vi "NI 9260 Synchronization 9230 (Host).vi"() -> ()   [LabVIEW 2021]
uses:
  <vilib>/LabVIEW Targets/FPGA/cRIO/shared/nicrio_ModuleControls/nicrio_cRIO-9260_DataRatesRing2.ctl
  <vilib>/LabVIEW Targets/FPGA/cRIO/shared/nicrio_ModuleControls/nicrio_cRIO-9230_DataRatesRing2.ctl
  <vilib>/FPGAPlugInAG/cRIO-9053/niLvFpga_Open_cRIO-9053.vi
  <vilib>/rvi/interface/common/dynamic/niFpgaDynamicAddResources.vi
  <vilib>/Utility/error.llb/Error Cluster From Error Code.vi
  <vilib>/rvi/errors/niLvFpgaAdjustHostInterfaceError.vi
  <vilib>/rvi/interface/common/niFpgaWaitOnOcc.vi
  <vilib>/FPGAPlugInAG/Dynamic/niLvFpga_Run_Dynamic.vi
  <vilib>/FPGAPlugInAG/Dynamic/niLvFpga_Close_Dynamic.vi
  <vilib>/rvi/interface/nirviOpenFPGA/nirviOpenFPGA.xnode
  FPGA Bitfiles/crio-ni9260_FPGATarget_NI9260Synchroniz_8mHRFd2dl5A.lvbitx
  <vilib>/rvi/interface/nirviReadWriteControl/nirviReadWriteControl.xnode
  <vilib>/rvi/interface/nirviMethod/nirviMethod.xnode
  <vilib>/rvi/interface/nirviCloseFPGA/nirviCloseFPGA.xnode
  <vilib>/rvi/interface/Simulation/niFpgaSimulationCallBeginRW.vi
  <vilib>/FPGAPlugInAG/Dynamic/niLvFpga_WriteFifo_Dynamic.vi
  <vilib>/rvi/errors/niLvFpgaMergeErrorWithErrorCode.vi
  <vilib>/FPGAPlugInAG/Dynamic/niLvFpga_ConfigureFifo_Dynamic.vi
  NiFpgaLv.dll
  <vilib>/FPGAPlugInAG/Dynamic/niLvFpga_ReadFifo_Dynamic.vi
panel:
  out "host rate (ms)":u32=80
  in  "Waveform":T1(ring)=enum."Square Wave"
  in  "NI 9230 Data Rate":T2=10 items=["12.800 kS/s (NI 9230)"=10, "11.378 kS/s (NI 9230)"=36, "10.240 kS/s (NI 9230)"=21, "9.309 kS/s (NI 9230)"=44, "8.533 kS/s (NI 9230)"=14, "7.877 kS/s (NI 9230)"=52, "7.314 kS/s (NI 9230)"=29, "6.827 kS/s (NI 9230)"=60, "6.400 kS/s (NI 9230)"=18, "6.024 kS/s (NI 9230)"=68, "5.689 kS/s (NI 9230)"=37, "5.389 kS/s (NI 9230)"=76, "5.120 kS/s (NI 9230)"=22, "4.876 kS/s (NI 9230)"=84, "4.655 kS/s (NI 9230)"=45, "4.452 kS/s (NI 9230)"=92, "4.267 kS/s (NI 9230)"=26, "4.096 kS/s (NI 9230)"=100, "3.938 kS/s (NI 9230)"=53, "3.657 kS/s (NI 9230)"=30, "3.413 kS/s (NI 9230)"=61, "3.200 kS/s (NI 9230)"=34, "3.012 kS/s (NI 9230)"=69, "2.844 kS/s (NI 9230)"=38, "2.695 kS/s (NI 9230)"=77, "2.560 kS/s (NI 9230)"=42, "2.438 kS/s (NI 9230)"=85, "2.327 kS/s (NI 9230)"=46, "2.226 kS/s (NI 9230)"=93, "2.133 kS/s (NI 9230)"=50, "2.048 kS/s (NI 9230)"=101, "1.969 kS/s (NI 9230)"=54, "1.829 kS/s (NI 9230)"=58, "1.707 kS/s (NI 9230)"=62, "1.600 kS/s (NI 9230)"=66, "1.506 kS/s (NI 9230)"=70, "1.422 kS/s (NI 9230)"=74, "1.347 kS/s (NI 9230)"=78, "1.280 kS/s (NI 9230)"=82, "1.219 kS/s (NI 9230)"=86, "1.164 kS/s (NI 9230)"=90, "1.113 kS/s (NI 9230)"=94, "1.067 kS/s (NI 9230)"=98, "1.024 kS/s (NI 9230)"=102, "0.985 kS/s (NI 9230)"=106]
  in  "NI 9260 Data Rate":T3=4 items=["51.200 kS/s (NI 9260)"=1, "25.600 kS/s (NI 9260)"=2, "17.067 kS/s (NI 9260)"=3, "12.800 kS/s (NI 9260)"=4, "10.240 kS/s (NI 9260)"=5, "8.533 kS/s (NI 9260)"=6, "7.314 kS/s (NI 9260)"=7, "6.400 kS/s (NI 9260)"=8, "5.689 kS/s (NI 9260)"=9, "5.120 kS/s (NI 9260)"=10, "4.654 kS/s (NI 9260)"=11, "4.267 kS/s (NI 9260)"=12, "3.938 kS/s (NI 9260)"=13, "3.657 kS/s (NI 9260)"=14, "3.413 kS/s (NI 9260)"=15, "3.200 kS/s (NI 9260)"=16, "3.012 kS/s (NI 9260)"=17, "2.845 kS/s (NI 9260)"=18, "2.695 kS/s (NI 9260)"=19, "2.560 kS/s (NI 9260)"=20, "2.438 kS/s (NI 9260)"=21, "2.328 kS/s (NI 9260)"=22, "2.226 kS/s (NI 9260)"=23, "2.133 kS/s (NI 9260)"=24, "2.048 kS/s (NI 9260)"=25, "1.969 kS/s (NI 9260)"=26, "1.896 kS/s (NI 9260)"=27, "1.829 kS/s (NI 9260)"=28, "1.765 kS/s (NI 9260)"=29, "1.707 kS/s (NI 9260)"=30, "1.652 kS/s (NI 9260)"=31]
  out "Analog Input":waveform(dbl)[](graph)=[{"t0"=timestamp(0 s since 1904-01-01), "dt"=7.8125e-05, "Y"=array[1024 elements]}, {"t0"=timestamp(0 s since 1904-01-01), "dt"=7.8125e-05, "Y"=array[1024 elements]}]
  out "NI 9230 FIFO Time Out":bool
  in  "Host Loop Rate (ms)":u32=1
  out "NI 9260 FIFO Time Out":bool
  in  "Waveform Settings":T4(array[cluster])=[{"Frequency (Hz)"=800.0, "Amplitude (V)"=2.5, "Offset (V)"=0.0, "Phase (deg)"=0.0}, {"Frequency (Hz)"=800.0, "Amplitude (V)"=2.5, "Offset (V)"=0.0, "Phase (deg)"=0.0}]
  in  "stop":bool
  out "FPGA Error out":errorcluster
  in  "Number of Samples per channel":dbl=1024.0 format="%.4p"
  out "Analog Output":waveform(dbl)[](graph)=[{"t0"=timestamp(0 s since 1904-01-01), "dt"=7.8125e-05, "Y"=array[1024 elements]}, {"t0"=timestamp(0.08 s since 1904-01-01), "dt"=7.8125e-05, "Y"=array[1024 elements]}]
  out "Host Error out":errorcluster
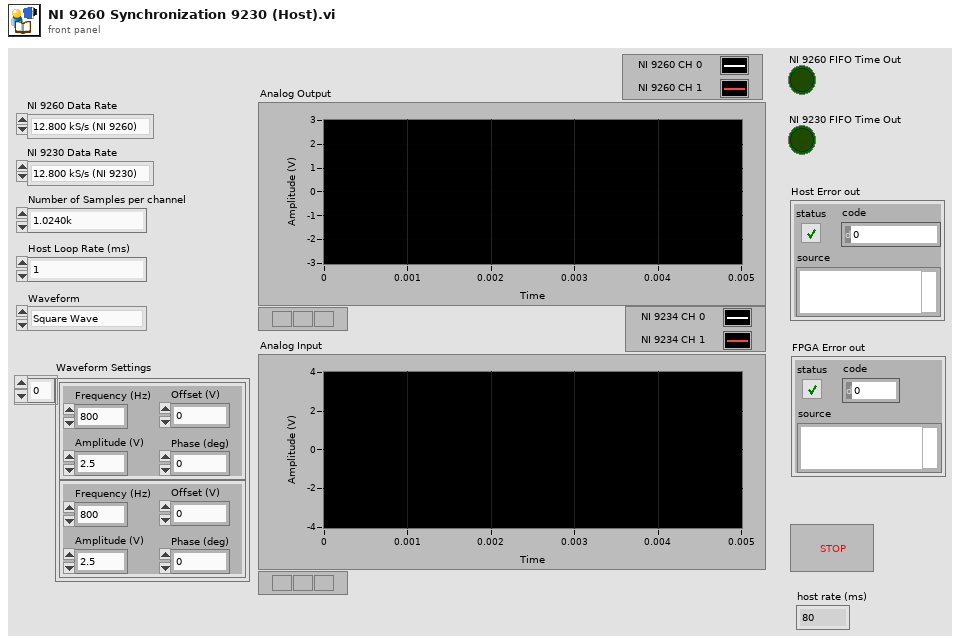
[diagram p1: front panel]
types:
  T1 = enum16{"Sawtooth Wave", "Square Wave", "Sine Wave"}
  T2 = typedef "nicrio_cRIO-9230_DataRatesRing2.ctl" = u8
  T3 = typedef "nicrio_cRIO-9260_DataRatesRing2.ctl" = u8
  T4 = cluster{"Frequency (Hz)":dbl, "Amplitude (V)":dbl, "Offset (V)":dbl, "Phase (deg)":dbl}[]
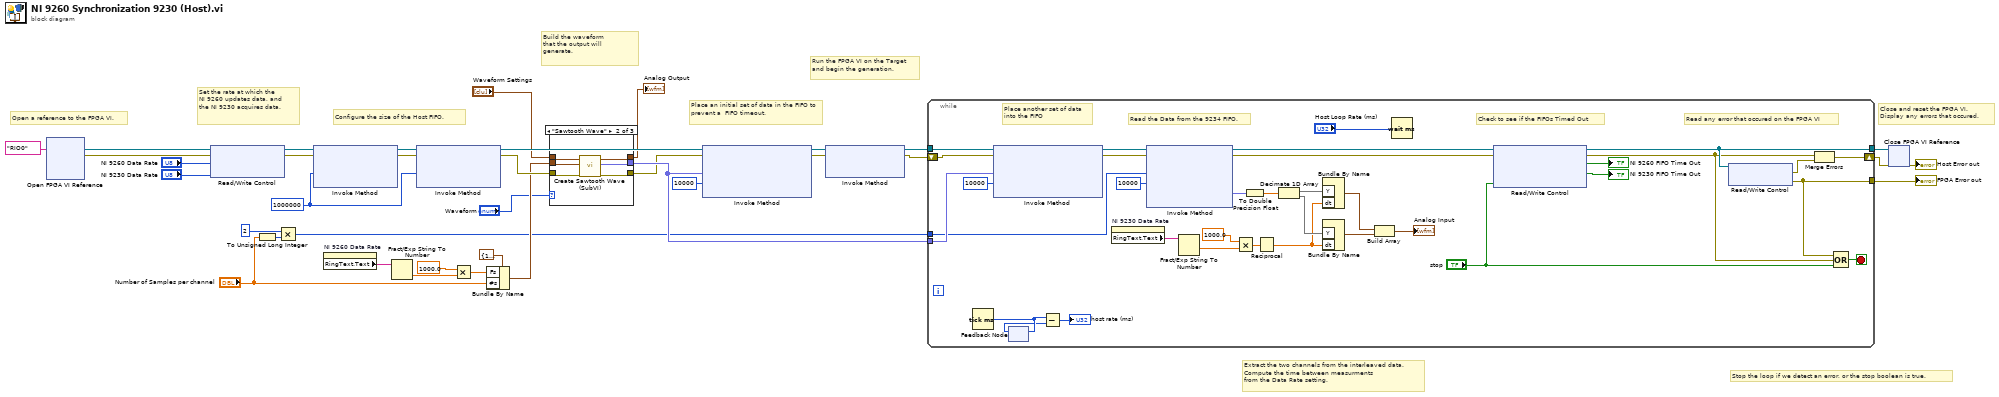
[diagram p0: block diagram]
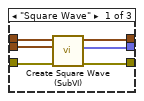
[diagram p2: hidden frame]
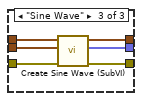
[diagram p3: hidden frame]
diagram:
  w2 = u32 1000000 ("Requested Depth")
  # "Build the waveform \nthat the output will generate."
  # "Extract the two channels from the interleaved data.\nCompute the time between measurments \nfrom the Data Rate setting."
  # "Place an initial set of data in the FIFO to prevent a  FIFO timeout."
  # "Stop the loop if we detect an error, or the stop boolean is true."
  # "Configure the size of the Host FIFO."
  # "Set the rate at which the \nNI 9260 updates data, and\nthe NI 9230 acquires data."
  # "Close and reset the FPGA VI. \nDisplay any errors that occured."
  # "Run the FPGA VI on the Target and begin the generation."
  # "Open a reference to the FPGA VI."
  n1 = xnode "Open FPGA VI Reference"("resource name"=tag "RIO0") -> ("FPGA VI Reference Out"=w34:refnum<k20>, "error out"=w36:errorcluster)  [unwired: 1 in]
  n2 = xnode "Read/Write Control"("FPGA VI Reference In"=w34, "error in"=w36, "NI 9260 Data Rate"="NI 9260 Data Rate", "NI 9230 Data Rate"="NI 9230 Data Rate") -> ("FPGA VI Reference Out"=w16:refnum<k20>, "error out"=w24:errorcluster)
  n3 = To Unsigned Long Integer(number="Number of Samples per channel") -> (unsigned 32bit integer=w29:u32)
  n4 = Multiply(x=u32 2, y=w29) -> (x*y=w3:u32)
  n5 = xnode "Invoke Method"("FPGA VI Reference In"=w16, "error in"=w24, "Requested Depth"=w2) -> ("FPGA VI Reference Out"=w15:refnum<k20>, "error out"=w17:errorcluster)  [unwired: 1 out]
  n6 = property on="NI 9260 Data Rate" class="Ring (strict)"() -> ("RingText.Text"=w5:string)  [unwired: 2 in, 2 out]
  n7 = Fract/Exp String To Number(string=w5) -> (number=w32:dbl)  [unwired: 3 in, 1 out]
  n8 = xnode "Invoke Method"("FPGA VI Reference In"=w15, "error in"=w17, "Requested Depth"=w2) -> ("FPGA VI Reference Out"=w26:refnum<k20>, "error out"=w14:errorcluster)  [unwired: 1 out]
  n9 = Multiply(x=1000.0, y=w32) -> (x*y=w21:dbl)
  n10 = Bundle By Name(cluster=cluster{"Fs":dbl, "#s":dbl} {"Fs"=1000.0, "#s"=1000.0} ("sampling info"), "Fs"=w21, "#s"="Number of Samples per channel") -> (w12:cluster{"Fs":dbl, "#s":dbl})
  n11 = case shown="\"Sawtooth Wave\"" "Waveform" {
    tunnel: w14 -> [w40 w46 w54]
    tunnel: "Waveform Settings" -> [w42 w48 w53]
    tunnel: w12 -> [w41 w47 w52]
    tunnel: [w37 w43 w51] -> w11
    tunnel: [w39 w44 w50] -> w10
    tunnel: [w38 w45 w49] -> w8
    frame "Square Wave" {
      n12 = call "Create Square Wave (SubVI).vi"("error in (no error)"=w40, "sampling info"=w41, "Sine Waveform Settings"=w42) -> ("error out"=w39:errorcluster, "FXP Sinewave"=w37:fxp<+/-,24,4>[], "Voltage Output Waveform"=w38:waveform(dbl)[])  [unwired: 6 in]
    }
    frame "Sawtooth Wave" {
      n13 = call "Create Sawtooth Wave (SubVI).vi"("error in (no error)"=w46, "sampling info"=w47, "Sine Waveform Settings"=w48) -> ("error out"=w44:errorcluster, "FXP Sinewave"=w43:fxp<+/-,24,4>[], "Voltage Output Waveform"=w45:waveform(dbl)[])  [unwired: 6 in]
    }
    frame "Sine Wave" {
      n14 = call "Create Sine Wave (SubVI).vi"("error in (no error)"=w54, "sampling info"=w52, "Sine Waveform Settings"=w53) -> ("error out"=w50:errorcluster, "FXP Sinewave"=w51:fxp<+/-,24,4>[], "Voltage Output Waveform"=w49:waveform(dbl)[])  [unwired: 6 in]
    }
  }
  "Analog Output" <- w8
  n15 = xnode "Invoke Method"("FPGA VI Reference In"=w26, "error in"=w10, "Data"=w11, "Timeout (ms)"=10000) -> ("FPGA VI Reference Out"=w25:refnum<k20>, "error out"=w27:errorcluster)  [unwired: 1 out]
  n16 = xnode "Invoke Method"("FPGA VI Reference In"=w25, "error in"=w27) -> ("FPGA VI Reference Out"=w28:refnum<k20>, "error out"=w9:errorcluster)  [unwired: 1 in]
  n17 = while {
    tunnel: w28 -> [w89]
    tunnel: w11 -> [w88]
    tunnel: [w78] -> w22
    tunnel: [w84] -> w18
    shift-right: [w66] -> w31
    shift-left: w9 -> [w64]
    tunnel: w3 -> [w57]
    stop <- w86 stop-if-true
    # "Check to see if the FIFOs Timed Out"
    # "Read any error that occured on the FPGA VI"
    # "Read the Data from the 9234 FIFO."
    # "Place another set of data\ninto the FIFO"
    n18 = Tick Count (ms)() -> (millisecond timer value=w56:u32)
    n19 = xnode "Invoke Method"("FPGA VI Reference In"=w89, "error in"=w64, "Data"=w88, "Timeout (ms)"=10000) -> ("FPGA VI Reference Out"=w83:refnum<k20>, "error out"=w82:errorcluster)  [unwired: 1 out]
    n20 = feedback-in #1(w56) -> ()
    n21 = feedback #1() -> (w55:u32)  [unwired: 1 in]
    n22 = Subtract(x=w56, y=w55) -> (x-y=→"host rate (ms)":u32)
    n23 = property on="NI 9230 Data Rate" class="Ring (strict)"() -> ("RingText.Text"=w61:string)  [unwired: 2 in, 2 out]
    n24 = xnode "Invoke Method"("FPGA VI Reference In"=w83, "error in"=w82, "Number of Elements"=w57, "Timeout (ms)"=10000) -> ("FPGA VI Reference Out"=w80:refnum<k20>, "error out"=w79:errorcluster, "Data"=w77:fxp<+/-,24,7>[])  [unwired: 1 out]
    n25 = Fract/Exp String To Number(string=w61) -> (number=w74:dbl)  [unwired: 4 out]
    n26 = Multiply(x=1000.0, y=w74) -> (x*y=w75:dbl)
    n27 = To Double Precision Float(number=w77) -> (double precision float=w67:dbl[])
    n28 = Reciprocal(x=w75) -> (1/x=w59:dbl)
    n29 = Decimate 1D Array(w67) -> (w71:dbl[], w60:dbl[])
    n30 = Bundle By Name("Y"=w71, "dt"=w59) -> (w73:waveform(dbl))  [unwired: 1 out]
    n31 = Bundle By Name("Y"=w60, "dt"=w59) -> (w72:waveform(dbl))  [unwired: 1 out]
    n32 = Build Array(w73, w72) -> (→"Analog Input":waveform(dbl)[])
    n33 = Wait (ms)(milliseconds to wait="Host Loop Rate (ms)") -> ()  [unwired: 1 out]
    n34 = xnode "Read/Write Control"("FPGA VI Reference In"=w80, "error in"=w79, "stop"="stop") -> ("FPGA VI Reference Out"=w78:refnum<k20>, "error out"=w65:errorcluster, "NI 9260 FIFO Time Out"=→"NI 9260 FIFO Time Out":bool, "NI 9230 FIFO Time Out"=→"NI 9230 FIFO Time Out":bool)
    n35 = xnode "Read/Write Control"("FPGA VI Reference In"=w78) -> ("error out"=w63:errorcluster, "FPGA Error out"=w84:errorcluster)  [unwired: 1 in, 1 out]
    n36 = Merge Errors(w65, w63) -> (w66:errorcluster)
    n37 = Compound Arithmetic op=OR(w84, w65, "stop") -> (w86:bool)
  }
  "FPGA Error out" <- w18
  n38 = xnode "Close FPGA VI Reference"("FPGA VI Reference In"=w22, "error in"=w31) -> ("error out"=→"Host Error out":errorcluster)
